vi "testLEDs.vi"() -> ()   [LabVIEW 2017]
panel:
  in  "Baud Rate":u32=115200
  in  "Value to write":i8
  in  "OK Button":bool
  out "LED state":bool[](array[boolean])
  in  "stop":bool
  in  "Arduino":refnum<visa-resource-name>
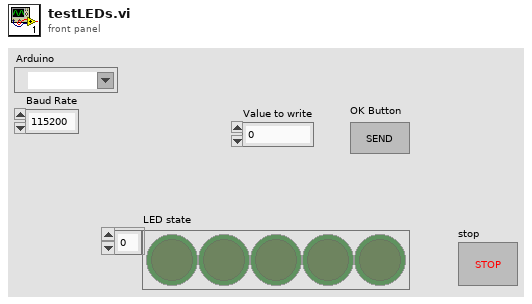
[diagram p1: front panel]
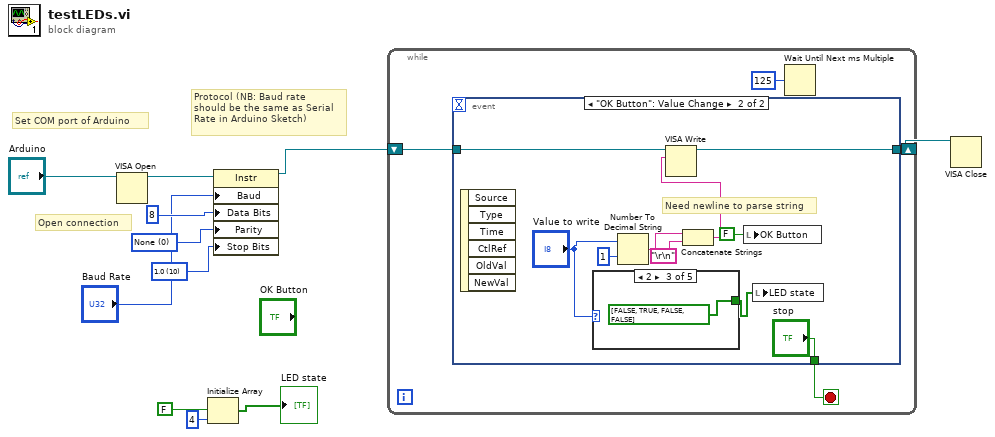
[diagram p0: block diagram]
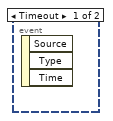
[diagram p2: hidden frame]
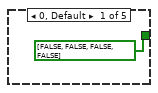
[diagram p3: hidden frame]
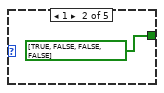
[diagram p4: hidden frame]
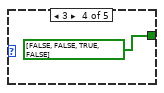
[diagram p5: hidden frame]
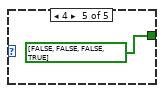
[diagram p6: hidden frame]
diagram:
  w7 = u16 0 items=["None", "Odd", "Even", "Mark", "Space"] ("Serial Settings:Parity")
  w8 = u16 10 items=["1.0"=10, "1.5"=15, "2.0"=20] ("Serial Settings:Stop Bits")
  # "Protocol (NB: Baud rate\nshould be the same as Serial \nRate in Arduino Sketch)"
  # "Open connection"
  # "Set COM port of Arduino"
  n1 = VISA Open(VISA resource name="Arduino") -> (VISA resource name=w10:refnum<visa-resource-name>)  [unwired: 4 in, 1 out]
  n2 = Initialize Array(FALSE, 4 ("dimension size")) -> (→"LED state":bool[])
  n3 = property class="Instr"(reference=w10, "Baud"="Baud Rate", "Data Bits"=u16 8 ("Serial Settings:Data Bits"), "Parity"=w7, "Stop Bits"=w8) -> (reference out=w3:refnum<visa-resource-name>)  [unwired: 1 in, 1 out]
  n4 = while {
    shift-right: [w13] -> w2
    shift-left: w3 -> [w14]
    stop <- w12 stop-if-true
    n5 = event shown="[1] \"OK Button\": Value Change" {
      selector: _ -> [_ _]
      dyn-events: _ -> [_ _]
      timeout: _ -> [_ _]
      tunnel: w14 -> [_ w25]
      tunnel: [_ w23] -> w13
      tunnel: [_ "stop"] -> w12
      event Timeout {
        n6 = event-data() -> ()  [unwired: 1 in, 3 out]
      }
      event "OK Button": Value Change {
        # "Need newline to parse string"
        n7 = event-data() -> ()  [unwired: 1 in, 6 out]
        n8 = case shown="2" "Value to write" {
          tunnel: [bool[] [FALSE, FALSE, FALSE, FALSE] bool[] [TRUE, FALSE, FALSE, FALSE] bool[] [FALSE, TRUE, FALSE, FALSE] bool[] [FALSE, FALSE, TRUE, FALSE] bool[] [FALSE, FALSE, FALSE, TRUE]] -> w21
          frame 0, Default {
          }
          frame 1 {
          }
          frame 2 {
          }
          frame 3 {
          }
          frame 4 {
          }
        }
        n9 = Number To Decimal String(number="Value to write", width (-)=i16 1) -> (decimal integer string=w20:string)
        n10 = Concatenate Strings(w20, "\r\n") -> (w19:string)
        n11 = VISA Write(VISA resource name=w25, write buffer=w19) -> (VISA resource name out=w23:refnum<visa-resource-name>)  [unwired: 1 in, 2 out]
        n12 = local write "OK Button"(FALSE ("OK Button")) -> ()
        n13 = local write "LED state"(w21) -> ()
      }
    }
    n14 = Wait Until Next ms Multiple(millisecond multiple=u32 125) -> ()  [unwired: 1 out]
  }
  n15 = VISA Close(VISA resource name=w2) -> ()  [unwired: 1 in, 1 out]
